vi "LWXPS_XYZGroupPositionPCORawEncoderGet.vi"(0 "XPS Reference IN":refnum<k24>, 5 "XYZ group name":string, 7 "Position X":dbl, 9 "Position Y":dbl, 11 "Position Z":dbl, 12 "LabVIEW error IN":errorcluster) -> (3 "XPS Reference OUT":refnum<k24>, 4 "Returned error code":i32, 6 "PCO Raw position X":dbl, 8 "PCO Raw position Y":dbl, 10 "PCO Raw position Z":dbl, 14 "LabVIEW error OUT":errorcluster, 15 "XPS Error String":string)   [LabVIEW 2014]
uses:
  D:/XPSQ8_LabView_Library/Development/Source/Dll/Newport.XPS.CommandInterface.dll
  Dll/Newport.XPS.CommandInterface.dll
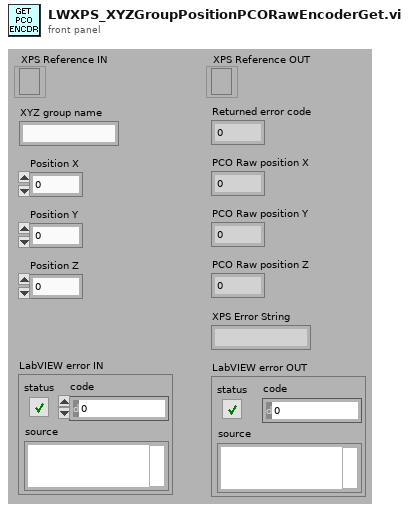
[diagram p1: front panel]
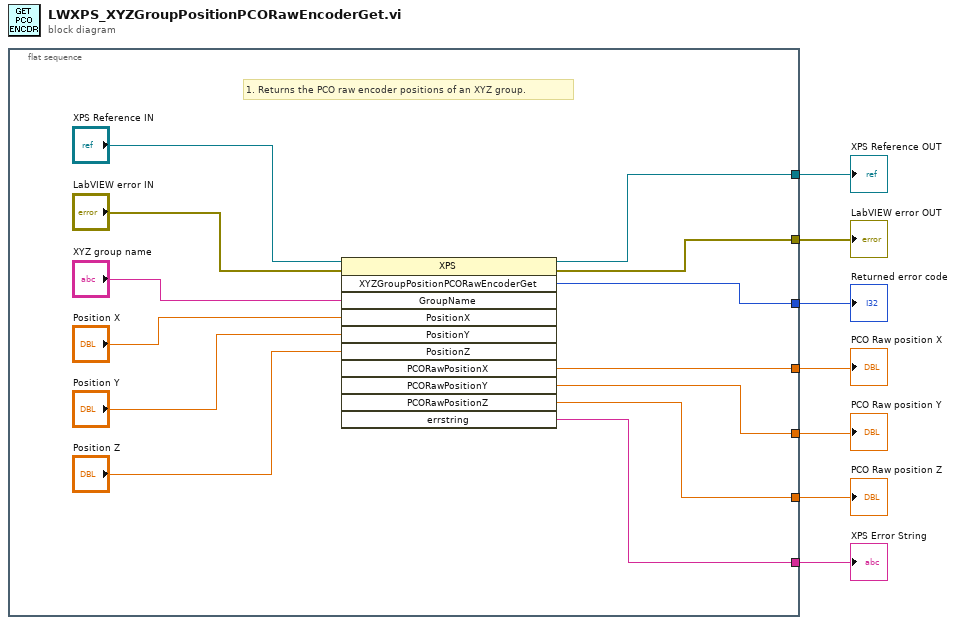
[diagram p0: block diagram]
diagram:
  n1 = flat-sequence {
    tunnel: [w18] -> w7
    tunnel: [w15] -> w6
    tunnel: [w19] -> w5
    tunnel: [w13] -> w1
    tunnel: [w8] -> w2
    tunnel: [w10] -> w3
    tunnel: [w9] -> w4
    frame #0 {
      # "1. Returns the PCO raw encoder positions of an XYZ group."
      n2 = invoke class="XPS" method="XYZGroupPositionPCORawEncoderGet"(reference="XPS Reference IN", error in="LabVIEW error IN", "GroupName"="XYZ group name", "PositionX"="Position X", "PositionY"="Position Y", "PositionZ"="Position Z") -> (reference out=w18:refnum<k24>, error out=w15:errorcluster, "XYZGroupPositionPCORawEncoderGet"=w19:i32, "PCORawPositionX"=w13:dbl, "PCORawPositionY"=w8:dbl, "PCORawPositionZ"=w10:dbl, "errstring"=w9:string)  [unwired: 5 in, 4 out]
    }
  }
  "XPS Reference OUT" <- w7
  "LabVIEW error OUT" <- w6
  "Returned error code" <- w5
  "XPS Error String" <- w4
  "PCO Raw position X" <- w1
  "PCO Raw position Y" <- w2
  "PCO Raw position Z" <- w3
